vi "set range.vi"() -> ()   [LabVIEW 2012]
panel:
  in  "auto scale":bool=TRUE caption="auto scale 2"
  in  "channel1":cluster{i32, i32}(slide)={0, 4096} scale=0.0..2047.0
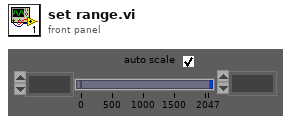
[diagram p1: front panel]
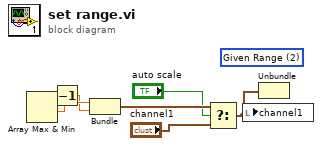
[diagram p0: block diagram]
diagram:
  w7 = u32 2 items=["Full Dynamic", "Downshift", "Given Range", "90% Dynamic", "Given Percent Range"] ("16-bit Display Mapping:Conversion Method")
  n1 = Array Max & Min() -> (max value=w4:dbl, min value=w5:dbl)  [unwired: 1 in, 2 out]
  n2 = Decrement(x=w4) -> (x-1=w3:dbl)
  n3 = Bundle(w5, w3) -> (w10:cluster{dbl, dbl})  [unwired: 1 in]
  n4 = Select(t=w10, s="auto scale", f="channel1") -> (s? t:f=w6:cluster{dbl, dbl})
  n5 = local write "channel1"(w6) -> ()
  n6 = Unbundle(w6) -> (w2:dbl, w1:dbl)
